vi "Remove ClientID Session.vi"(8 "error in (no error)":errorcluster, 10 "SessionMailbox":refnum<queue>, 11 "MQTT Server":refnum<class "Server.lvclass">) -> (0 "error out":errorcluster, 3 "MQTT Server":refnum<class "Server.lvclass">)   [LabVIEW 2013, in "MQTT Server.lvlib" / "Server.lvclass"]
uses:
  Server.lvclass
  MQTT_Base/Base Class/Response -- cluster.ctl
  <vilib>/LabVIEW Open Source Project/MQTT Control Packets/Control Packets/ControlPacket/ControlPacket.lvclass
  Server.lvclass/Server.ctl
  MQTT_Base/Base Class/MQTT_Base.lvclass
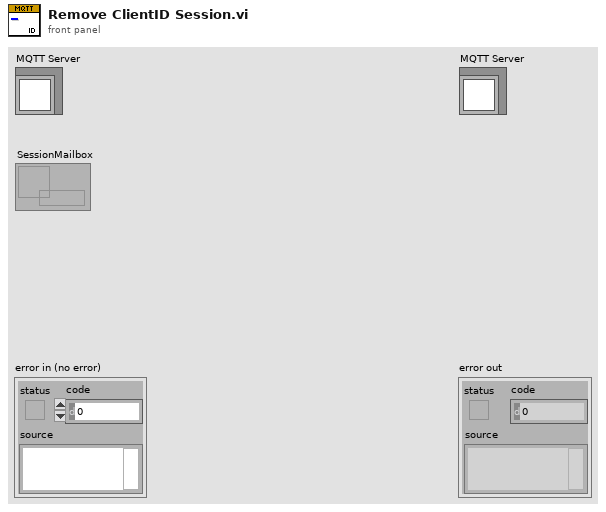
[diagram p1: front panel]
types:
  T1 = typedef "MQTT Server.lvlib/Server.lvclass/SessionRef -- cluster.ctl" = cluster{"ClientID":string, "SessionMailbox":refnum<queue>}
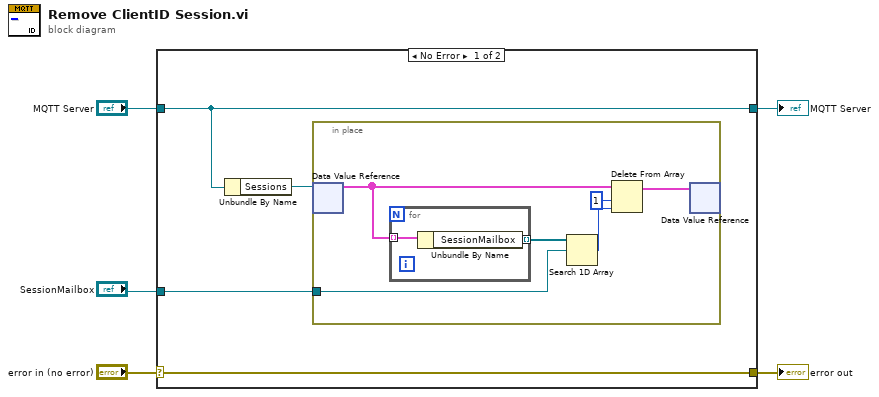
[diagram p0: block diagram]
diagram:
  n1 = case shown="No Error" "error in (no error)" {
    selector: "error in (no error)" -> [w6 w19]
    tunnel: [w6 w19] -> w4
    tunnel: [w8 w18] -> w2
    tunnel: "MQTT Server" -> [w8 w18]
    tunnel: "SessionMailbox" -> [w7 _]
    frame No Error {
      n2 = Unbundle By Name(w8) -> ("Sessions"=w9:refnum<data-value>)
      n3 = in-place {
        in-place-border: w7 -> [w14]
        n4 = in-place-dvr #1(w9) -> (w13:T1[])  [unwired: 1 out]
        n5 = for {
          tunnel: w13 -> [w17] mode=indexing
          tunnel: [w16] -> w15 mode=indexing
          n6 = Unbundle By Name(w17) -> ("SessionMailbox"=w16:refnum<queue>)
        }
        n7 = Search 1D Array(1D array=w15, element=w14) -> (index of element=w11:i32)  [unwired: 1 in]
        n8 = Delete From Array(array=w13, length=1, index=w11) -> (array with subset deleted=w10:T1[])  [unwired: 1 out]
        n9 = in-place-dvr #1(w10) -> ()  [unwired: 2 out]
      }
    }
    frame Error {
    }
  }
  "error out" <- w4
  "MQTT Server" <- w2
